vi "Parse Comment-Text.vi"(8 "Error In":errorcluster) -> (0 "Error Out":errorcluster)   [LabVIEW 2018, in "Tests.lvlib" / "Parser.lvlib"]
uses:
  Parser.lvlib
  src/Toolkit/Public/Tokens/Text/Text.lvclass
  src/Toolkit/Public/Readers/Public/String/String.lvclass
  D:/Users/cfield/Code/Field R&D Services/Mustache/trunk/src/Mustache/Public/Readers/Public/Abstract/Abstract.lvclass
  <vilib>/Utility/LVClass/Get LV Class Name.vi
  src/Toolkit/Public/Tokens/Text/API/Read Content.vi
  <vilib>/addons/_JKI Toolkits/Caraya/classes/Assert/Assert Equal_Variant.vi
  <vilib>/addons/_JKI Toolkits/Caraya/classes/Test/Test.lvclass
  src/Toolkit/Public/Parser/Parser.lvclass
  <vilib>/addons/_JKI Toolkits/Caraya/classes/Assert/Assert.lvclass
  Tests.lvlib
  src/Toolkit/Public/Tokens/Abstract/Abstract.lvclass
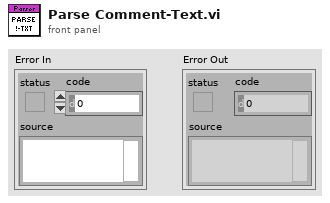
[diagram p1: front panel]
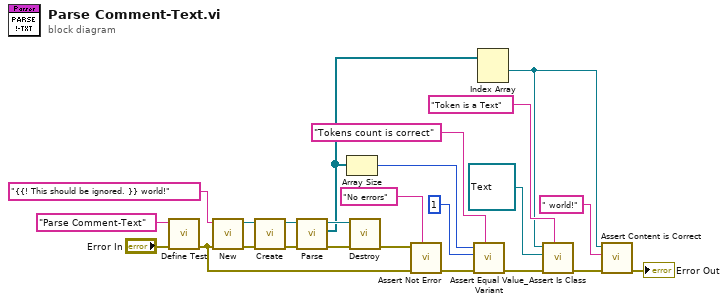
[diagram p0: block diagram]
diagram:
  n1 = call <vilib>:"Define Test.vi"("error in (no error)"="Error In", "Label (VI Title)"="Parse Comment-Text") -> ("error out"=w15:errorcluster)  [unwired: 9 in]
  n2 = call "New.vi"("Error In"=w15, "String"="{{! This should be ignored. }} world!" ("format string")) -> ("Error Out"=w21:errorcluster, "String"=w22:refnum<class "String.lvclass">)  [unwired: 8 in]
  n3 = call "Create.vi"("Error In"=w21, "Reader"=w22) -> ("Error Out"=w20:errorcluster, "Parser"=w19:refnum<class "Parser.lvclass">)  [unwired: 8 in]
  n4 = call "Parse.vi"("Error In"=w20, "Parser In"=w19) -> ("Error Out"=w17:errorcluster, "Tokens"=w9:refnum<class "Abstract.lvclass">[], "Parser Out"=w18:refnum<class "Parser.lvclass">)  [unwired: 7 in]
  n5 = Array Size(array=w9) -> (size(s)=w11:i32)
  n6 = call "Destroy.vi"("Error In"=w17, "Parser"=w18) -> ("Error Out"=w16:errorcluster)  [unwired: 9 in]
  n7 = call <vilib>:"Assert Not Error.vi"("Label"="No errors", "error in (no error)"=w15, "Not Error?"=w16) -> ("error out"=w13:errorcluster)  [unwired: 8 in]
  n8 = call <vilib>:"Assert Equal Value_Variant.vi"("Label"="Tokens count is correct", "error in (no error)"=w13, "Y"=1 ("size(s)"), "X"=w11) -> ("error out"=w5:errorcluster)  [unwired: 7 in]
  n9 = Index Array(array=w9) -> (element #1=w1:refnum<class "Abstract.lvclass">)  [unwired: 2 in, 1 out]
  n10 = call "Assert Is Class.vi"("Label"="Token is a Text", "Error In"=w5, "Expected"=refnum<class "Text.lvclass"> refnum ("Mustache.lvlib:Tokens.lvlib:Text.lvclass"), "Actual"=w1) -> ("Error Out"=w7:errorcluster)  [unwired: 7 in]
  n11 = call "Assert Content is Correct.vi"("Error In"=w7, "Expected"=" world!", "Token"=w1) -> ("Error Out"=→"Error Out":errorcluster)  [unwired: 8 in]
